vi "isHomed-Old-Controllers.vi"(3 "Motor (XYZ)":string(combo)="X", 5 "Device in":refnum<k24>) -> (2 "Device out":refnum<k24>)   [LabVIEW 2014]
doc: "André Romero - 2017\nandretec@ifsc.usp.br"
uses:
  C:/user-Lab/AndreTec/GITs/andretec/Thorlabs-Vector-Move/kinesisTec/Kinesis/Thorlabs.MotionControl.TCube.DCServoCLI.dll
  kinesisTec/Kinesis/Thorlabs.MotionControl.TCube.DCServoCLI.dll
  C:/user-Lab/AndreTec/GITs/andretec/Thorlabs-Vector-Move/kinesisTec/Kinesis/Thorlabs.MotionControl.GenericMotorCLI.dll
  kinesisTec/Kinesis/Thorlabs.MotionControl.GenericMotorCLI.dll
  motor-XYZ-GlobalVar.vi
panel:
  out "IsHomed":bool
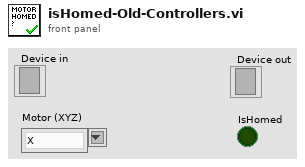
[diagram p1: front panel]
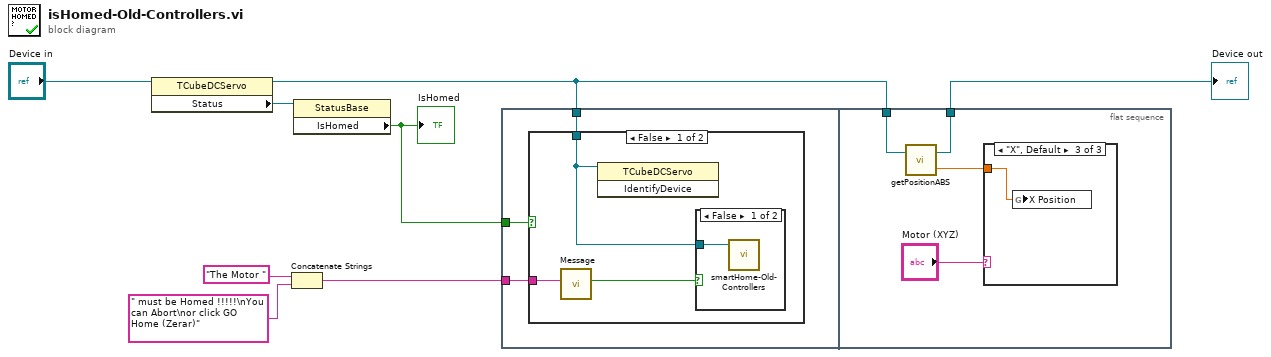
[diagram p0: block diagram]
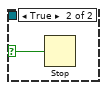
[diagram p2: hidden frame]
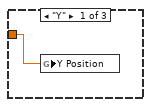
[diagram p4: hidden frame]
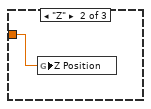
[diagram p5: hidden frame]
diagram:
  n1 = property class="TCubeDCServo"(reference="Device in") -> (reference out=w2:refnum<k24>, "Status"=w7:refnum<k24>)  [unwired: 1 in, 1 out]
  n2 = Concatenate Strings("The Motor ", " must be Homed !!!!!\nYou can Abort\nor click GO Home (Zerar)" ("string")) -> (w5:string)
  n3 = property class="StatusBase"(reference=w7) -> ("IsHomed"=w8:bool)  [unwired: 1 in, 2 out]
  "IsHomed" <- w8
  n4 = flat-sequence {
    tunnel: w8 -> [w11]
    tunnel: w5 -> [w10]
    tunnel: w2 -> [w9]
    tunnel: w2 -> [w20]
    tunnel: [w19] -> w1
    frame #0 {
      n5 = case shown="False" w11 {
        tunnel: w10 -> [w14 _]
        tunnel: w9 -> [w12 _]
        frame False {
          n6 = call "Message"("Message"=w14) -> ("Abort"=w13:bool)  [unwired: 9 in, 1 out]
          n7 = invoke class="TCubeDCServo" method="IdentifyDevice"(reference=w12) -> ()  [unwired: 2 in, 3 out]
          n8 = case shown="False" w13 {
            selector: w13 -> [_ w16]
            tunnel: w12 -> [w15 _]
            frame False {
              n9 = call "smartHome-Old-Controllers.vi"("Device in"=w15) -> ()  [unwired: 4 in, 1 out]
            }
            frame True {
              n10 = Stop(stop? (T)=w16) -> ()
            }
          }
        }
        frame True {
        }
      }
    }
    frame #1 {
      n11 = call "getPositionABS.vi"("Device"=w20) -> ("GetPOS"=w18:dbl, "Device out"=w19:refnum<k24>)  [unwired: 1 in]
      n12 = case shown="\"X\", Default" "Motor (XYZ)" {
        tunnel: w18 -> [w21 w22 w23]
        frame "Y" {
          n13 = global write "motor-XYZ-GlobalVar.vi" "Y Position"(w21) -> ()
        }
        frame "Z" {
          n14 = global write "motor-XYZ-GlobalVar.vi" "Z Position"(w22) -> ()
        }
        frame "X", Default {
          n15 = global write "motor-XYZ-GlobalVar.vi" "X Position"(w23) -> ()
        }
      }
    }
  }
  "Device out" <- w1
